vi "TEMP_VI.vi"(8 "stop":bool, 11 "COM Bluegiga in":refnum<visa-resource-name>="COM13") -> (0 "Reading":bool, 1 "Numeric":dbl, 2 "Text":string caption="Result", 3 "Connected":bool)   [LabVIEW 2020]
uses:
  <vilib>/BLE/type_def/connection_status_bundle.ctl
  <vilib>/BLE/type_def/address_type.ctl
panel:
  out "MAC Address":string
  out "Handle table":string[][](array[string])
  out "Connection Status":T1={"MAC Address"="", "cnx handle"=0, "cnx flags"=0, "Address Type"=125, "Connection Interval (ms)"=125, "Timeout(ms)"=125, "Latency"=0, "bonding handle"=0} {"Address Type" items=["Public", "Random"]}
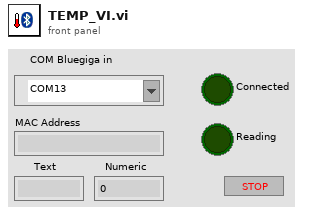
[diagram p1: front panel]
types:
  T1 = typedef "connection_status_bundle.ctl" = cluster{"MAC Address":string, "cnx handle":u8, "cnx flags":u8, "Address Type":T2, "Connection Interval (ms)":u16, "Timeout(ms)":u16, "Latency":u16, "bonding handle":u8}
  T2 = typedef "address_type.ctl" = u8
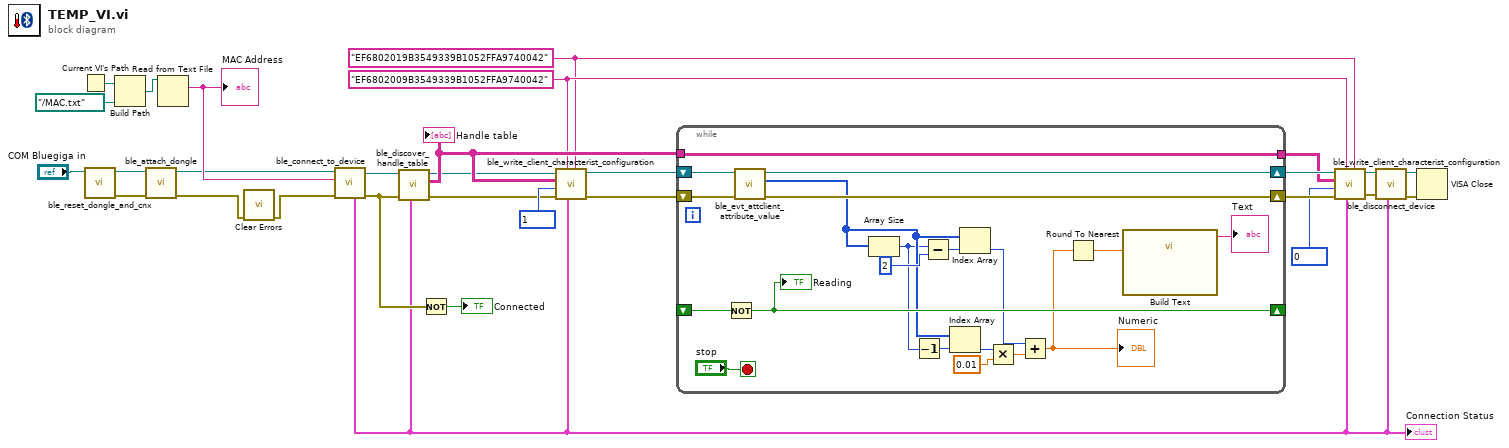
[diagram p0: block diagram]
diagram:
  w2 = "EF6802009B3549339B1052FFA9740042"
  w1 = "EF6802019B3549339B1052FFA9740042"
  n1 = Current VI's Path() -> (path=w6:path)
  n2 = call <vilib>:"ble_reset_dongle_and_cnx.vi"("COM Bluegiga in"="COM Bluegiga in") -> ("error out"=w28:errorcluster, "COM Bluegiga out"=w26:refnum<visa-resource-name>)  [unwired: 9 in]
  n3 = Build Path(base path=w6, name or relative path=path "../MAC.txt") -> (appended path=w7:path)
  n4 = call <vilib>:"ble_attach_dongle.vi"("error in (no error)"=w28, "COM Bluegiga in"=w26) -> ("error out"=w4:errorcluster, "COM Bluegiga out"=w5:refnum<visa-resource-name>)  [unwired: 8 in]
  n5 = Read from Text File(file (use dialog)=w7) -> (text=w9:string)  [unwired: 3 in, 3 out]
  "MAC Address" <- w9
  n6 = call <vilib>:"Clear Errors.vi"("error in (no error)"=w4) -> ("error out"=w10:errorcluster)  [unwired: 5 in, 1 out]
  n7 = call <vilib>:"ble_connect_to_device.vi"("error in (no error)"=w10, "MAC Address"=w9, "COM Bluegiga in"=w5) -> ("error out"=w24:errorcluster, "COM Bluegiga out"=w25:refnum<visa-resource-name>, "Connection Status"=w18:T1)  [unwired: 6 in]
  "Connection Status" <- w18
  n8 = call <vilib>:"ble_discover_handle_table.vi"("Connection Status"=w18, "error in (no error)"=w24, "COM Bluegiga in"=w25) -> ("error out"=w13:errorcluster, "Handle table"=w15:string[][], "COM Bluegiga out"=w14:refnum<visa-resource-name>)  [unwired: 6 in]
  "Handle table" <- w15
  n9 = Not(x=w24) -> (.not. x?=→"Connected":bool)
  n10 = call <vilib>:"ble_write_client_characterist_configuration.vi"("Characteristic UUID"=w1, "Connection Status"=w18, "Service UUID"=w2, "error in (no error)"=w13, "Value(16bit)"=u16 1, "Handle table"=w15, "COM Bluegiga in"=w14) -> ("error out"=w11:errorcluster, "COM Bluegiga out"=w12:refnum<visa-resource-name>)  [unwired: 3 in]
  n11 = while {
    tunnel: w15 -> [w45]
    shift-right: [w48] -> w22
    shift-left: w12 -> [w50]
    shift-right: [w44] -> w23
    shift-left: w11 -> [w49]
    tunnel: [w45] -> w21
    shift-right: [w47] -> _
    shift-left: _ -> [w46]
    stop <- "stop" stop-if-true
    n12 = Not(x=w46) -> (.not. x?=w47:bool)
    "Reading" <- w47
    n13 = call <vilib>:"ble_evt_attclient_attribute_value.vi"("error in (no error)"=w49, "COM Bluegiga in"=w50) -> ("error out"=w44:errorcluster, "characteristic value"=w39:u8[], "COM Bluegiga out"=w48:refnum<visa-resource-name>)  [unwired: 6 in, 1 out]
    n14 = Array Size(array=w39) -> (size(s)=w37:i32)
    n15 = Decrement(x=w37) -> (x-1=w38:i32)
    n16 = Subtract(x=w37, y=2) -> (x-y=w42:i32)
    n17 = Index Array(array=w39, index=w38) -> (element=w36:u8)
    n18 = Index Array(array=w39, index=w42) -> (element=w33:u8)
    n19 = Multiply(x=w36, y=0.01) -> (x*y=w34:dbl)
    n20 = Add(x=w33, y=w34) -> (x+y=w31:dbl)
    "Numeric" <- w31
    n21 = Round To Nearest(number=w31) -> (nearest integer value=w32:dbl)
    n22 = call "Build Text"("T"=w32) -> ("Result"=→"Text":string)  [unwired: 13 in, 1 out]
  }
  n23 = call <vilib>:"ble_write_client_characterist_configuration.vi"("Characteristic UUID"=w1, "Connection Status"=w18, "Service UUID"=w2, "error in (no error)"=w23, "Value(16bit)"=u16 0, "Handle table"=w21, "COM Bluegiga in"=w22) -> ("error out"=w19:errorcluster, "COM Bluegiga out"=w20:refnum<visa-resource-name>)  [unwired: 3 in]
  n24 = call <vilib>:"ble_disconnect_device.vi"("Connection Status"=w18, "error in (no error)"=w19, "COM Bluegiga in"=w20) -> ("error out"=w29:errorcluster, "COM Bluegiga out"=w30:refnum<visa-resource-name>)  [unwired: 7 in]
  n25 = VISA Close(VISA resource name=w30, error in (no error)=w29) -> ()  [unwired: 1 out]
